vi "quiz GPS (2).vi"(0 "TRAMA":string) -> (1 "Arreglo salida RMC":string[](array[string]), 2 "Arreglo salida GGA":string[](array[string]), 3 "Arreglo salida GSA":string[](array[string]))   [LabVIEW 2020]
doc: "Este sub vi, recibe una trama GP### y la decodifica retornando el valor de la fecha, hora y velocidad."
panel:
  out "VDOP":string
  out "HDOP":string
  out "PDOP":string
  out "Satellite usado 12":string
  out "Satellite usado 11":string
  out "Satellite usado 10":string
  out "Satellite usado 9":string
  out "Satellite usado 8":string
  out "Satellite usado 7":string
  out "Satellite usado 6":string
  out "Satellite usado 5":string
  out "Satellite usado 4":string
  out "Satellite usado 3":string
  out "Satellite usado 2":string
  out "Satellite usado 1":string
  out "Fix status (GSA)":string
  out "MODE":string
  out "Cheksum data (GSA)":string
  out "Cheksum data (GGA)":string
  out "DGPS station ID":string
  out "DGPS AGE (seconds)":string
  out "Geoid Separation(Metros)":string
  out "Altitud(M = metros)":string
  out "HDOP":string
  out "Num satelites usados":string
  out "Longitud (GGA)":string
  out "Latitud (GGA)":string
  out "Variación magnetica":string
  out "Angulo en degrees":string
  out "Longitud":string
  out "Latitud":string
  out "Data valid":string
  out "Fix status":string
  out "di":string
  out "Dirección lat(GGA)":string
  out "Estado de trama":bool
  out "Positioning mode":string
  out "Cheksum data":string
  out "Dir":string
  out "d":string
  out "Dirección":string
  out "hora (GGA)":string
  out "Velocidad en knots":string
  out "Fecha\ndd/mm/yy":string
  out "Hora\nhh/mm/ssss":string
  # "RMC"
  # "N = No fix\nA = Autonomous GNSS fix\nD = Differential GNSS fix"
  # "GGA"
  # "0 = Invalid\n1 = GNSS fix\n2 = DGPS fix\n6 = Estimated (dead reckoning) mode"
  # "GSA"
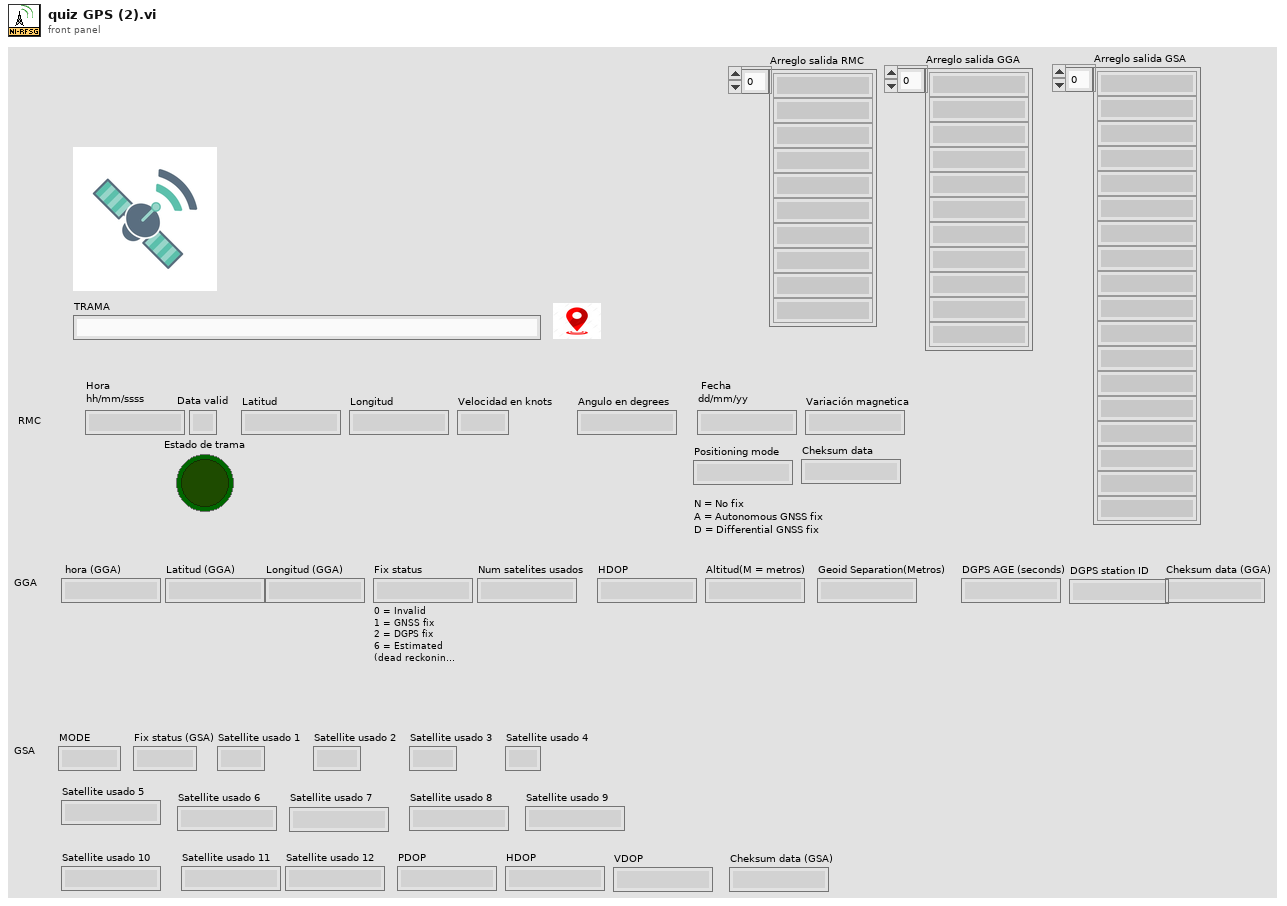
[diagram p1: front panel]
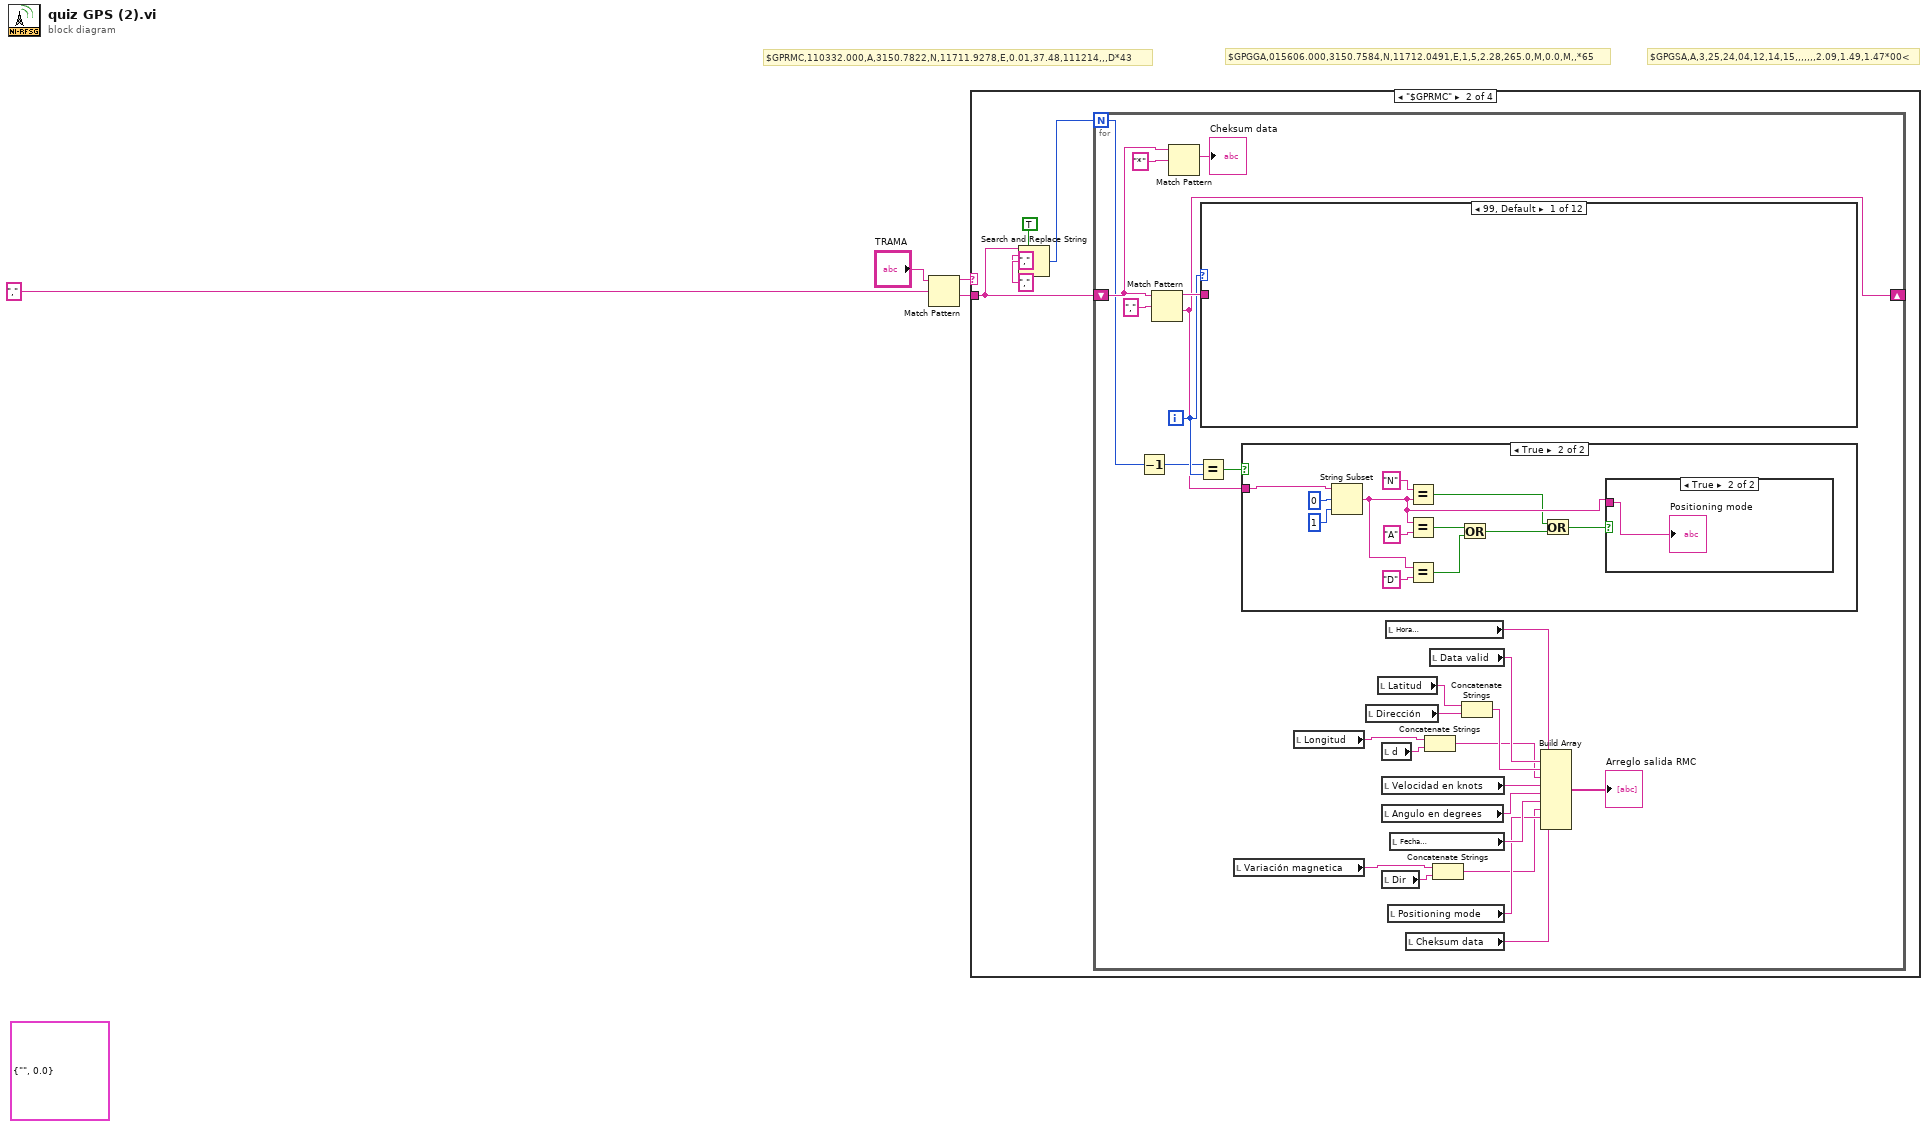
[diagram p0: block diagram]
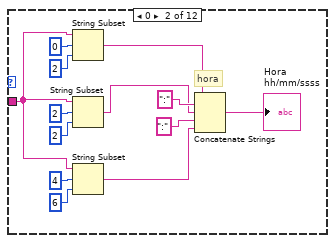
[diagram p5: hidden frame]
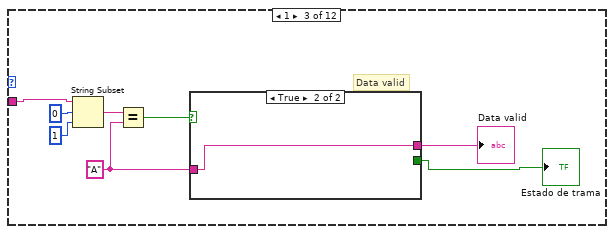
[diagram p6: hidden frame]
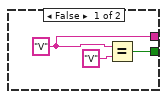
[diagram p7: hidden frame]
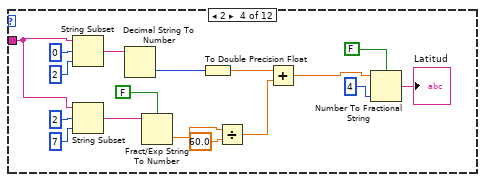
[diagram p8: hidden frame]
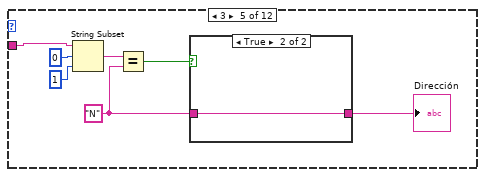
[diagram p9: hidden frame]
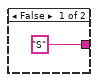
[diagram p10: hidden frame]
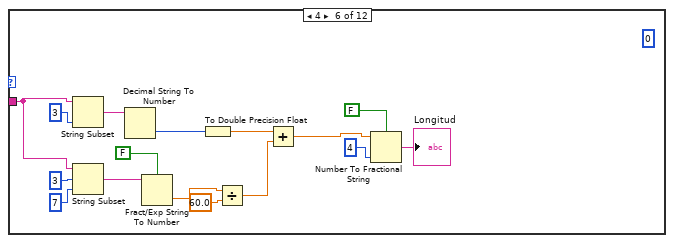
[diagram p11: hidden frame]
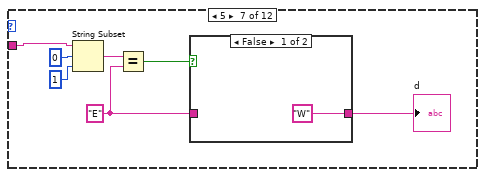
[diagram p12: hidden frame]
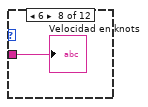
[diagram p14: hidden frame]
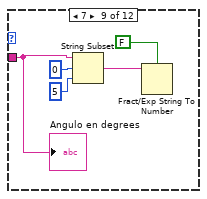
[diagram p15: hidden frame]
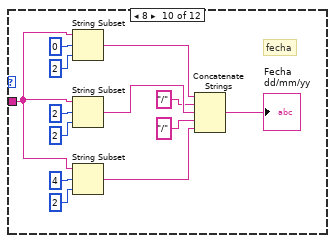
[diagram p16: hidden frame]
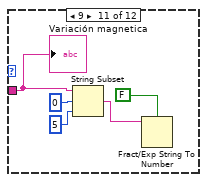
[diagram p17: hidden frame]
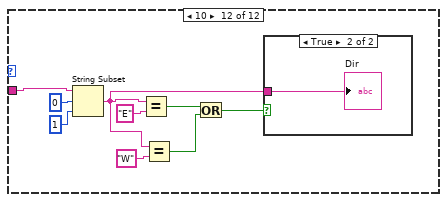
[diagram p18: hidden frame]
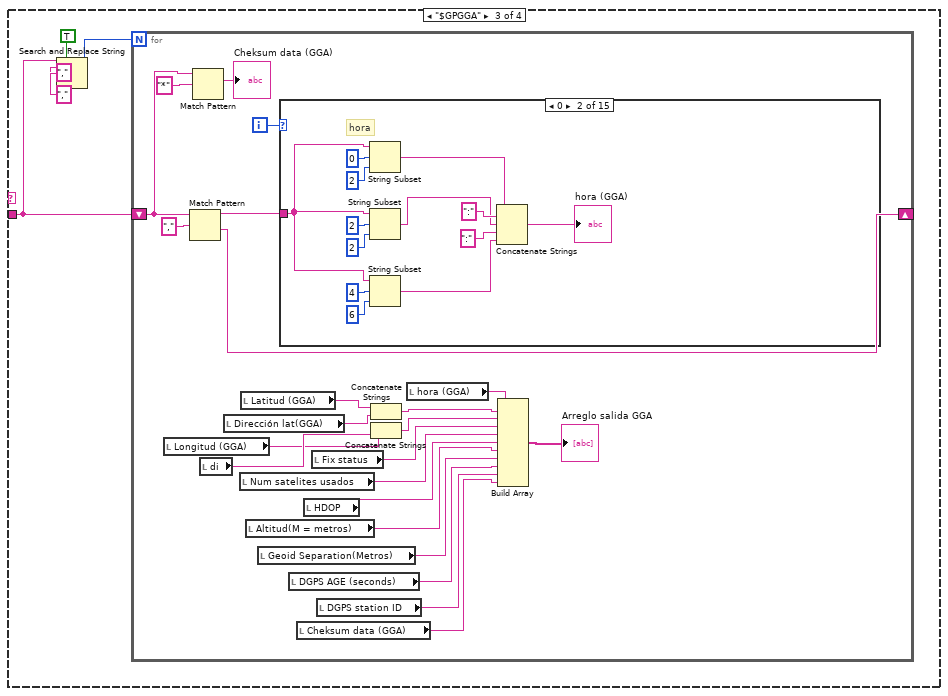
[diagram p20: hidden frame]
diagram:
  (unwired) cluster{string, dbl} {"", 0.0}
  # "$GPGSA,A,3,25,24,04,12,14,15,,,,,,,2.09,1.49,1.47*00<"
  # "$GPGGA,015606.000,3150.7584,N,11712.0491,E,1,5,2.28,265.0,M,0.0,M,,*65"
  # "$GPRMC,110332.000,A,3150.7822,N,11711.9278,E,0.01,37.48,111214,,,D*43"
  n1 = Match Pattern(string="TRAMA", regular expression=",") -> (before substring=w2:string, after substring=w1:string)  [unwired: 1 in, 2 out]
  n2 = case shown="\"$GPRMC\"" w2 {
    tunnel: w1 -> [_ w6 w160 w281]
    frame "False", Default {
    }
    frame "$GPRMC" {
      n3 = Search and Replace String(replace all?=TRUE ("replace all? (F)"), input string=w6, search string=",", replace string="," ("regular expression")) -> (number of replacements=w7:i32)  [unwired: 4 in, 3 out]
      n4 = for {
        N: w7 -> [w31]
        shift-right: [w28] -> _
        shift-left: w6 -> [w34]
        i -> [w32]
        n5 = Decrement(x=w31) -> (x-1=w30:i32)
        n6 = Match Pattern(string=w34, regular expression=",") -> (before substring=w35:string, after substring=w28:string)  [unwired: 1 in, 2 out]
        n7 = Match Pattern(string=w34, regular expression="*") -> (after substring=→"Cheksum data":string)  [unwired: 1 in, 3 out]
        n8 = Equal?(x=w30, y=w32) -> (x = y?=w29:bool)
        n9 = case shown="99, Default" w32 {
          tunnel: w35 -> [_ w60 w68 w79 w94 w105 w119 w126 w127 w133 w145 w156]
          frame 99, Default {
          }
          frame 0 {
            # "hora"
            n10 = String Subset(string=w60, offset (0)=0, length (rest)=2 ("length (rest)")) -> (substring=w53:string)
            n11 = String Subset(string=w60, offset (0)=2, length (rest)=2 ("length (rest)")) -> (substring=w52:string)
            n12 = String Subset(string=w60, offset (0)=4, length (rest)=6 ("length (rest)")) -> (substring=w51:string)
            n13 = Concatenate Strings(w53, ":" ("string"), w52, ":" ("string"), w51) -> (→"Hora\nhh/mm/ssss":string)
          }
          frame 1 {
            w64 = "A"
            # "Data valid"
            n14 = String Subset(string=w68, offset (0)=0, length (rest)=1 ("length (rest)")) -> (substring=w69:string)
            n15 = Equal?(x=w69, y=w64) -> (x = y?=w66:bool)
            n16 = case shown="True" w66 {
              tunnel: [w72 _] -> w65
              tunnel: w64 -> [_ w74]
              tunnel: [w71 w74] -> w63
              frame False {
                w71 = "V" ("Fecha")
                n17 = Equal?(x=w71, y="V") -> (x = y?=w72:bool)
              }
              frame True {
              }
            }
            "Estado de trama" <- w65
            "Data valid" <- w63
          }
          frame 2 {
            n18 = String Subset(string=w79, offset (0)=0, length (rest)=2) -> (substring=w89:string)
            n19 = String Subset(string=w79, offset (0)=2, length (rest)=7) -> (substring=w81:string)
            n20 = Decimal String To Number(string=w89) -> (number=w86:i32)  [unwired: 2 in, 1 out]
            n21 = Fract/Exp String To Number(use system decimal point (T)=FALSE, string=w81) -> (number=w80:dbl)  [unwired: 2 in, 1 out]
            n22 = To Double Precision Float(number=w86) -> (double precision float=w83:dbl)
            n23 = Divide(x=w80, y=60.0) -> (x/y=w84:dbl)
            n24 = Add(x=w83, y=w84) -> (x+y=w77:dbl)
            n25 = Number To Fractional String(use system decimal point (T)=FALSE, number=w77, precision (6)=i16 4) -> (F-format string=→"Latitud":string)  [unwired: 1 in]
          }
          frame 3 {
            w93 = "N"
            n26 = String Subset(string=w94, offset (0)=0, length (rest)=1 ("length (rest)")) -> (substring=w97:string)
            n27 = Equal?(x=w97, y=w93) -> (x = y?=w95:bool)
            n28 = case shown="True" w95 {
              tunnel: w93 -> [_ w100]
              tunnel: ["S" ("Fecha") w100] -> w92
              frame False {
              }
              frame True {
              }
            }
            "Dirección" <- w92
          }
          frame 4 {
            (unwired) 0
            n29 = String Subset(string=w105, length (rest)=3) -> (substring=w106:string)  [unwired: 1 in]
            n30 = String Subset(string=w105, offset (0)=3, length (rest)=7) -> (substring=w108:string)
            n31 = Decimal String To Number(string=w106) -> (number=w113:i32)  [unwired: 2 in, 1 out]
            n32 = Fract/Exp String To Number(use system decimal point (T)=FALSE, string=w108) -> (number=w107:dbl)  [unwired: 2 in, 1 out]
            n33 = To Double Precision Float(number=w113) -> (double precision float=w110:dbl)
            n34 = Divide(x=w107, y=60.0) -> (x/y=w111:dbl)
            n35 = Add(x=w110, y=w111) -> (x+y=w102:dbl)
            n36 = Number To Fractional String(use system decimal point (T)=FALSE, number=w102, precision (6)=i16 4) -> (F-format string=→"Longitud":string)  [unwired: 1 in]
          }
          frame 5 {
            w118 = "E"
            n37 = String Subset(string=w119, offset (0)=0, length (rest)=1 ("length (rest)")) -> (substring=w122:string)
            n38 = Equal?(x=w122, y=w118) -> (x = y?=w120:bool)
            n39 = case shown="False" w120 {
              tunnel: w118 -> [_ w125]
              tunnel: ["W" ("Fecha") w125] -> w117
              frame False {
              }
              frame True {
              }
            }
            "d" <- w117
          }
          frame 6 {
            "Velocidad en knots" <- w126
          }
          frame 7 {
            n40 = String Subset(string=w127, offset (0)=0, length (rest)=5) -> (substring=w128:string)
            n41 = Fract/Exp String To Number(use system decimal point (T)=FALSE, string=w128) -> ()  [unwired: 2 in, 2 out]
            "Angulo en degrees" <- w127
          }
          frame 8 {
            # "fecha"
            n42 = String Subset(string=w133, offset (0)=0, length (rest)=2 ("length (rest)")) -> (substring=w142:string)
            n43 = String Subset(string=w133, offset (0)=2, length (rest)=2 ("length (rest)")) -> (substring=w143:string)
            n44 = String Subset(string=w133, offset (0)=4, length (rest)=2 ("length (rest)")) -> (substring=w144:string)
            n45 = Concatenate Strings(w142, "/" ("string"), w143, "/" ("string"), w144) -> (→"Fecha\ndd/mm/yy":string)
          }
          frame 9 {
            n46 = String Subset(string=w145, offset (0)=0, length (rest)=5) -> (substring=w146:string)
            n47 = Fract/Exp String To Number(use system decimal point (T)=FALSE, string=w146) -> ()  [unwired: 2 in, 2 out]
            "Variación magnetica" <- w145
          }
          frame 10 {
            n48 = String Subset(string=w156, offset (0)=0, length (rest)=1 ("length (rest)")) -> (substring=w150:string)
            n49 = Equal?(x=w150, y="E") -> (x = y?=w153:bool)
            n50 = Equal?(x=w150, y="W" ("f")) -> (x = y?=w152:bool)
            n51 = Or(x=w153, y=w152) -> (x .or. y?=w151:bool)
            n52 = case shown="True" w151 {
              tunnel: w150 -> [_ w159]
              frame False {
              }
              frame True {
                "Dir" <- w159
              }
            }
          }
        }
        n53 = local read "Variación magnetica"() -> (w13:string)
        n54 = case shown="True" w29 {
          tunnel: w28 -> [_ w40]
          frame False {
          }
          frame True {
            n55 = String Subset(string=w40, offset (0)=0, length (rest)=1 ("length (rest)")) -> (substring=w41:string)
            n56 = Equal?(x="N" ("f"), y=w41) -> (x = y?=w38:bool)
            n57 = Equal?(x=w41, y="A" ("f")) -> (x = y?=w45:bool)
            n58 = Equal?(x=w41, y="D" ("f")) -> (x = y?=w44:bool)
            n59 = Or(x=w45, y=w44) -> (x .or. y?=w39:bool)
            n60 = Or(x=w38, y=w39) -> (x .or. y?=w37:bool)
            n61 = case shown="True" w37 {
              tunnel: w41 -> [_ w49]
              frame False {
              }
              frame True {
                "Positioning mode" <- w49
              }
            }
          }
        }
        n62 = local read "Longitud"() -> (w16:string)
        n63 = local read "Dirección"() -> (w18:string)
        n64 = local read "Latitud"() -> (w19:string)
        n65 = local read "d"() -> (w15:string)
        n66 = local read "Velocidad en knots"() -> (w25:string)
        n67 = local read "Angulo en degrees"() -> (w23:string)
        n68 = local read "Dir"() -> (w12:string)
        n69 = local read "Hora\nhh/mm/ssss"() -> (w27:string)
        n70 = local read "Positioning mode"() -> (w21:string)
        n71 = local read "Fecha\ndd/mm/yy"() -> (w22:string)
        n72 = local read "Cheksum data"() -> (w20:string)
        n73 = Concatenate Strings(w16, w15) -> (w14:string)
        n74 = local read "Data valid"() -> (w26:string)
        n75 = Concatenate Strings(w13, w12) -> (w11:string)
        n76 = Concatenate Strings(w19, w18) -> (w17:string)
        n77 = Build Array(w27, w26, w17, w14, w25, w23, w22, w11, w21, w20) -> (→"Arreglo salida RMC":string[])
      }
    }
    frame "$GPGGA" {
      n78 = Search and Replace String(replace all?=TRUE ("replace all? (F)"), input string=w160, search string=",", replace string="," ("regular expression")) -> (number of replacements=w162:i32)  [unwired: 4 in, 3 out]
      n79 = for {
        N: w162 -> [_]
        shift-right: [w186] -> _
        shift-left: w160 -> [w166]
        i -> [w184]
        n80 = local read "Longitud (GGA)"() -> (w177:string)
        n81 = Match Pattern(string=w166, regular expression=",") -> (before substring=w185:string, after substring=w186:string)  [unwired: 1 in, 2 out]
        n82 = Match Pattern(string=w166, regular expression="*") -> (after substring=→"Cheksum data (GGA)":string)  [unwired: 1 in, 3 out]
        n83 = local read "di"() -> (w178:string)
        n84 = local read "Dirección lat(GGA)"() -> (w180:string)
        n85 = local read "Num satelites usados"() -> (w174:string)
        n86 = local read "Latitud (GGA)"() -> (w181:string)
        n87 = local read "Altitud(M = metros)"() -> (w172:string)
        n88 = local read "Geoid Separation(Metros)"() -> (w171:string)
        n89 = case shown="0" w184 {
          tunnel: w185 -> [_ w198 w205 w219 w231 w244 w254 w268 w272 w275 _ w278 _ w279 w280]
          frame 99, Default {
          }
          frame 0 {
            # "hora"
            n90 = String Subset(string=w198, offset (0)=0, length (rest)=2 ("length (rest)")) -> (substring=w191:string)
            n91 = String Subset(string=w198, offset (0)=2, length (rest)=2 ("length (rest)")) -> (substring=w190:string)
            n92 = String Subset(string=w198, offset (0)=4, length (rest)=6 ("length (rest)")) -> (substring=w189:string)
            n93 = Concatenate Strings(w191, ":" ("string"), w190, ":" ("string"), w189) -> (→"hora (GGA)":string)
          }
          frame 1 {
            n94 = String Subset(string=w205, offset (0)=0, length (rest)=2) -> (substring=w215:string)
            n95 = String Subset(string=w205, offset (0)=2, length (rest)=7) -> (substring=w207:string)
            n96 = Decimal String To Number(string=w215) -> (number=w212:i32)  [unwired: 2 in, 1 out]
            n97 = Fract/Exp String To Number(use system decimal point (T)=FALSE, string=w207) -> (number=w206:dbl)  [unwired: 2 in, 1 out]
            n98 = To Double Precision Float(number=w212) -> (double precision float=w209:dbl)
            n99 = Divide(x=w206, y=60.0) -> (x/y=w210:dbl)
            n100 = Add(x=w209, y=w210) -> (x+y=w202:dbl)
            n101 = Number To Fractional String(use system decimal point (T)=FALSE, number=w202, precision (6)=i16 4) -> (F-format string=→"Latitud (GGA)":string)  [unwired: 1 in]
          }
          frame 2 {
            w220 = "N"
            n102 = String Subset(string=w219, offset (0)=0, length (rest)=1 ("length (rest)")) -> (substring=w223:string)
            n103 = Equal?(x=w223, y=w220) -> (x = y?=w221:bool)
            n104 = case shown="False" w221 {
              tunnel: w220 -> [_ w226]
              tunnel: ["S" ("Fecha") w226] -> w218
              frame False {
              }
              frame True {
              }
            }
            "Dirección lat(GGA)" <- w218
          }
          frame 3 {
            (unwired) 0
            n105 = String Subset(string=w231, length (rest)=3) -> (substring=w232:string)  [unwired: 1 in]
            n106 = String Subset(string=w231, offset (0)=3, length (rest)=7) -> (substring=w234:string)
            n107 = Decimal String To Number(string=w232) -> (number=w239:i32)  [unwired: 2 in, 1 out]
            n108 = Fract/Exp String To Number(use system decimal point (T)=FALSE, string=w234) -> (number=w233:dbl)  [unwired: 2 in, 1 out]
            n109 = To Double Precision Float(number=w239) -> (double precision float=w236:dbl)
            n110 = Divide(x=w233, y=60.0) -> (x/y=w237:dbl)
            n111 = Add(x=w236, y=w237) -> (x+y=w227:dbl)
            n112 = Number To Fractional String(use system decimal point (T)=FALSE, number=w227, precision (6)=i16 4) -> (F-format string=→"Longitud (GGA)":string)  [unwired: 1 in]
          }
          frame 4 {
            w245 = "E"
            n113 = String Subset(string=w244, offset (0)=0, length (rest)=1 ("length (rest)")) -> (substring=w248:string)
            n114 = Equal?(x=w248, y=w245) -> (x = y?=w246:bool)
            n115 = case shown="False" w246 {
              tunnel: w245 -> [_ w251]
              tunnel: ["W" ("Fecha") w251] -> w243
              frame False {
              }
              frame True {
              }
            }
            "di" <- w243
          }
          frame 5 {
            n116 = String Subset(string=w254, offset (0)=0, length (rest)=1 ("length (rest)")) -> (substring=w253:string)
            n117 = case shown="\"0\"" w253 {
              selector: w253 -> [_ w258 w259 w260 w261]
              tunnel: ["" w258 w259 w260 w261] -> w252
              frame "False", Default {
              }
              frame "0" {
              }
              frame "1" {
              }
              frame "2" {
              }
              frame "6" {
              }
            }
            "Fix status" <- w252
          }
          frame 6 {
            n118 = Decimal String To Number(string=w268) -> (number=w266:i32)  [unwired: 2 in, 1 out]
            n119 = Greater?(x=w266, y=0) -> (0:w263:bool)
            n120 = Less Or Equal?(x=w266, y=24) -> (x <= y?=w264:bool)
            n121 = And(x=w264, y=w263) -> (x .and. y?=w262:bool)
            n122 = case shown="False" w262 {
              tunnel: w268 -> [_ w271]
              tunnel: ["Error" w271] -> w267
              frame False {
              }
              frame True {
              }
            }
            "Num satelites usados" <- w267
          }
          frame 7 {
            "HDOP" <- w272
          }
          frame 8 {
            n123 = Concatenate Strings(w275, "M" ("string")) -> (→"Altitud(M = metros)":string)
          }
          frame 9 {
          }
          frame 10 {
            n124 = Concatenate Strings(w278, "M" ("string")) -> (→"Geoid Separation(Metros)":string)
          }
          frame 11 {
          }
          frame 12 {
            "DGPS AGE (seconds)" <- w279
          }
          frame 13 {
            "DGPS station ID" <- w280
          }
        }
        n125 = local read "DGPS AGE (seconds)"() -> (w170:string)
        n126 = local read "Cheksum data (GGA)"() -> (w165:string)
        n127 = local read "HDOP"() -> (w173:string)
        n128 = local read "Fix status"() -> (w175:string)
        n129 = local read "DGPS station ID"() -> (w169:string)
        n130 = Concatenate Strings(w181, w180) -> (w179:string)
        n131 = Concatenate Strings(w177, w178) -> (w176:string)
        n132 = local read "hora (GGA)"() -> (w183:string)
        n133 = Build Array(w183, w179, w176, w175, w174, w173, w172, w171, w170, w169, w165) -> (→"Arreglo salida GGA":string[])
      }
    }
    frame "$GPGSA" {
      n134 = Search and Replace String(replace all?=TRUE ("replace all? (F)"), input string=w281, search string=",", replace string="," ("regular expression")) -> (number of replacements=w282:i32)  [unwired: 4 in, 3 out]
      n135 = for {
        N: w282 -> [_]
        shift-right: [w308] -> _
        shift-left: w281 -> [w294]
        i -> [w307]
        n136 = Match Pattern(string=w294, regular expression=",") -> (before substring=w306:string, after substring=w308:string)  [unwired: 1 in, 2 out]
        n137 = Match Pattern(string=w294, regular expression="*") -> (after substring=→"Cheksum data (GSA)":string)  [unwired: 1 in, 3 out]
        n138 = case shown="15" w307 {
          tunnel: w306 -> [_ w312 w313 w314 w315 w316 w317 w318 w319 w320 w321 w322 w323 w324 w325 w326 w327 w328]
          frame 99, Default {
          }
          frame 0 {
            "MODE" <- w312
          }
          frame 1 {
            "Fix status (GSA)" <- w313
          }
          frame 2 {
            "Satellite usado 1" <- w314
          }
          frame 3 {
            "Satellite usado 2" <- w315
          }
          frame 4 {
            "Satellite usado 3" <- w316
          }
          frame 5 {
            "Satellite usado 4" <- w317
          }
          frame 6 {
            "Satellite usado 5" <- w318
          }
          frame 7 {
            "Satellite usado 6" <- w319
          }
          frame 8 {
            "Satellite usado 7" <- w320
          }
          frame 9 {
            "Satellite usado 8" <- w321
          }
          frame 10 {
            "Satellite usado 9" <- w322
          }
          frame 11 {
            "Satellite usado 10" <- w323
          }
          frame 12 {
            "Satellite usado 11" <- w324
          }
          frame 13 {
            "Satellite usado 12" <- w325
          }
          frame 14 {
            "PDOP" <- w326
          }
          frame 15 {
            "HDOP" <- w327
          }
          frame 16 {
            "VDOP" <- w328
          }
        }
        n139 = local read "Satellite usado 4"() -> (w300:string)
        n140 = local read "Satellite usado 3"() -> (w301:string)
        n141 = local read "Satellite usado 11"() -> (w291:string)
        n142 = local read "Satellite usado 2"() -> (w302:string)
        n143 = local read "Satellite usado 5"() -> (w299:string)
        n144 = local read "Satellite usado 9"() -> (w293:string)
        n145 = local read "Satellite usado 1"() -> (w303:string)
        n146 = local read "Fix status (GSA)"() -> (w304:string)
        n147 = local read "Cheksum data (GSA)"() -> (w286:string)
        n148 = local read "Satellite usado 12"() -> (w290:string)
        n149 = local read "Satellite usado 7"() -> (w297:string)
        n150 = local read "Satellite usado 10"() -> (w292:string)
        n151 = local read "Satellite usado 6"() -> (w298:string)
        n152 = local read "Satellite usado 8"() -> (w296:string)
        n153 = local read "VDOP"() -> (w287:string)
        n154 = local read "HDOP"() -> (w288:string)
        n155 = local read "PDOP"() -> (w289:string)
        n156 = local read "MODE"() -> (w305:string)
        n157 = Build Array(w305, w304, w303, w302, w301, w300, w299, w298, w297, w296, w293, w292, w291, w290, w289, w288, w287, w286) -> (→"Arreglo salida GSA":string[])
      }
    }
  }
